vi "LP Motor Loop Decide.vi"(8 "error in (no error)":errorcluster, 11 "Queue in":refnum<queue>) -> (0 "error out":errorcluster, 1 "Data":variant, 2 "CMD":T1, 3 "queue out":refnum<queue>)   [LabVIEW 2015]
uses:
  Stream/Controls/LP Motor CMD.ctl
  Stream/Controls/LP Motor Instruction.ctl
  Stream/LP Globals.vi
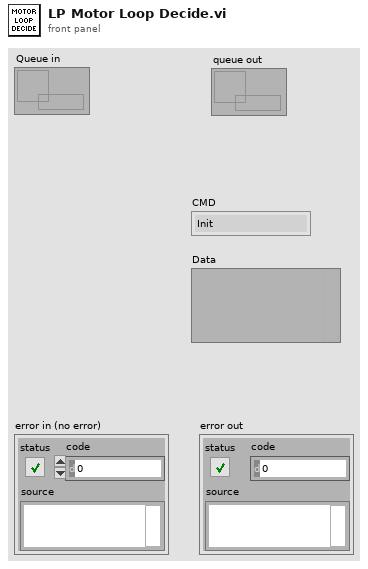
[diagram p1: front panel]
types:
  T1 = typedef "LP Motor CMD.ctl" = enum16{"Init", "SetAccelaration", "SetMaxVelocity", "Idle", "ClosedLoopRun", "MoveAbsolute", "MoveRelative", "MoveSRelative", "MoveSAbsolute", "StopMotors", "EnabeMotors", "SetZero", "StopMotion", "SetLoop", "FindHome", "MotorsGoToLimits", "ErrorHandling", "CloseMotor"}
  T2 = typedef "LP Motor Instruction.ctl" = cluster{"CMD":T1, "Data":variant}
  T3 = typedef "Motor Loop Mode Typedef.ctl" = enum16{"NotActive", "Open Loop", "Closed Loop", "ClosedOnce"}
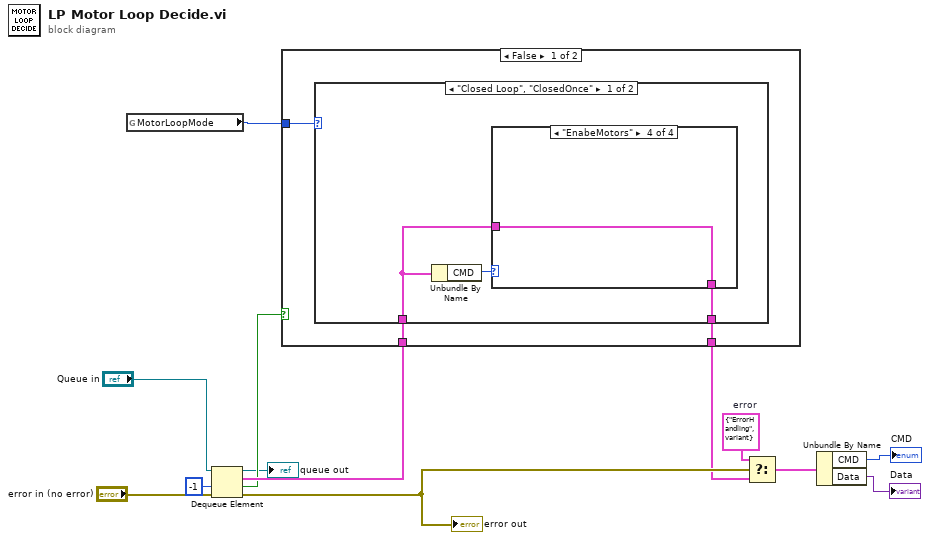
[diagram p0: block diagram]
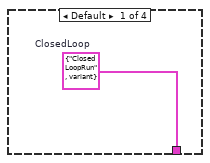
[diagram p2: hidden frame]
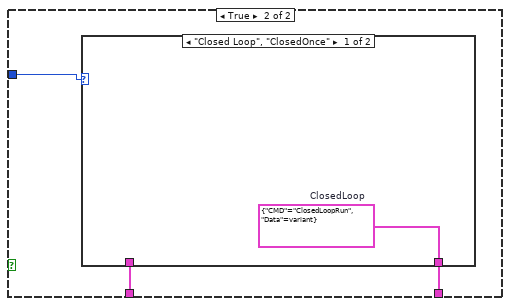
[diagram p6: hidden frame]
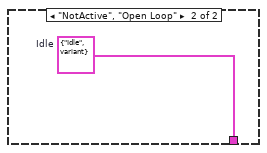
[diagram p7: hidden frame]
diagram:
  w8 = T2 {"CMD"=enum."ErrorHandling", "Data"=variant}  # error
  n1 = global read "LP Globals.vi" "MotorLoopMode"() -> (w6:T3)
  n2 = Dequeue Element(queue="Queue in", timeout in ms (-1)=-1, error in (no error)="error in (no error)") -> (queue out=→"queue out":refnum<queue>, element=w5:T2, timed out?=w3:bool, error out=w9:errorcluster)
  "error out" <- w9
  n3 = case shown="False" w3 {
    tunnel: w6 -> [w16 w27]
    tunnel: w5 -> [w15 w25]
    tunnel: [w14 w26] -> w4
    frame False {
      n4 = case shown="\"Closed Loop\", \"ClosedOnce\"" w16 {
        tunnel: w15 -> [w17 w24]
        tunnel: [w18 w24] -> w14
        frame "Closed Loop", "ClosedOnce" {
          n5 = Unbundle By Name(w17) -> ("CMD"=w19:T1)
          n6 = case shown="\"EnabeMotors\"" w19 {
            tunnel: [w20 w21 w22 w23] -> w18
            tunnel: w17 -> [_ w21 w22 w23]
            frame Default {
              w20 = T2 {"CMD"=enum."ClosedLoopRun", "Data"=variant}  # ClosedLoop
            }
            frame "StopMotors" {
            }
            frame "SetLoop" {
            }
            frame "EnabeMotors" {
            }
          }
        }
        frame "NotActive", "Open Loop" {
        }
      }
    }
    frame True {
      n7 = case shown="\"Closed Loop\", \"ClosedOnce\"" w27 {
        tunnel: [w28 w29] -> w26
        tunnel: w25 -> [_ _]
        frame "Closed Loop", "ClosedOnce" {
          w28 = T2 {"CMD"=enum."ClosedLoopRun", "Data"=variant}  # ClosedLoop
        }
        frame "NotActive", "Open Loop" {
          w29 = T2 {"CMD"=enum."Idle", "Data"=variant}  # Idle
        }
      }
    }
  }
  n8 = Select(t=w8, s=w9, f=w4) -> (s? t:f=w7:T2)
  n9 = Unbundle By Name(w7) -> ("CMD"=→"CMD":T1, "Data"=→"Data":variant)
